vi "EnFlo_Error_Handler.vi"(3 "error in (no error)":errorcluster, 4 "Error Type":string, 5 "Dialog Box (T)":bool=TRUE) -> (0 "Continue":bool, 1 "SMS Message":string, 2 "Email Message":string)   [LabVIEW 2014]
uses:
  Controls/Post_Process.ctl
  <vilib>/Utility/error.llb/DialogType.ctl
  Globals/Meas_global.vi
  Globals/Trav_pos_global.vi
  Globals/Preference_global.vi
  Email_transfer_global.vi
  Globals/Dynamic_call_global.ph.vi
panel:
  out "error out":errorcluster
  in  "Case Constant\n(See Context Help)":bool
  out "Server copy Location":path
  out "Hours Running":dbl format="%.2f"
  out "Error Information":string
  out "Log Files":path[](array[path])
  out "Frequency":i32
  out "Error Analysis":string
  out "Error Types":string[](array[string])
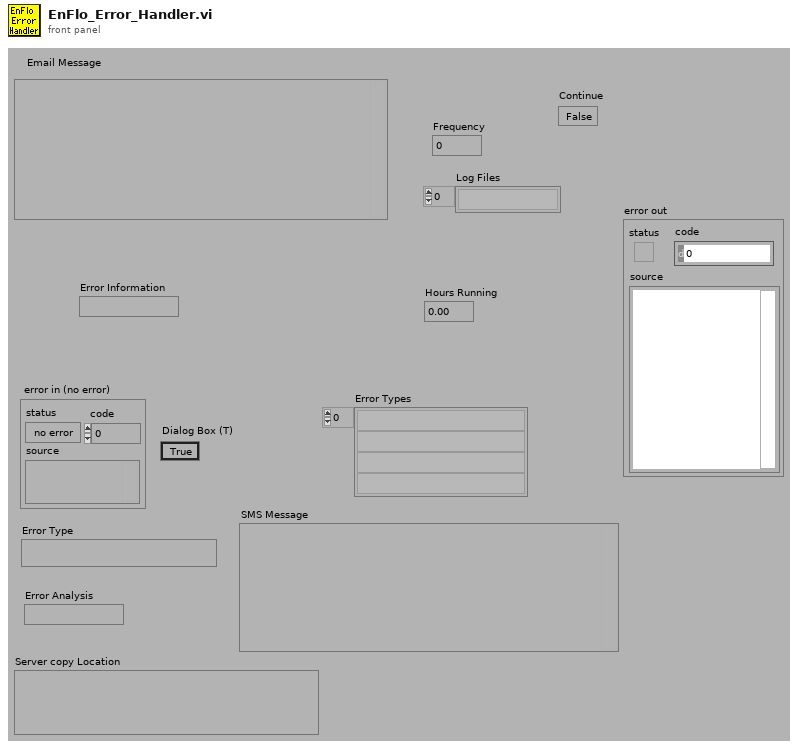
[diagram p1: front panel]
types:
  T1 = typedef "Post_Process.ctl" = enum16{"Take New Data", "Post Process Raw Data File"}
  T2 = cluster{"path":path, "data":string, "binary":bool, "MIME content-type \n(application/octet-stream)":string}[]
  T3 = typedef "DialogType.ctl" = u16
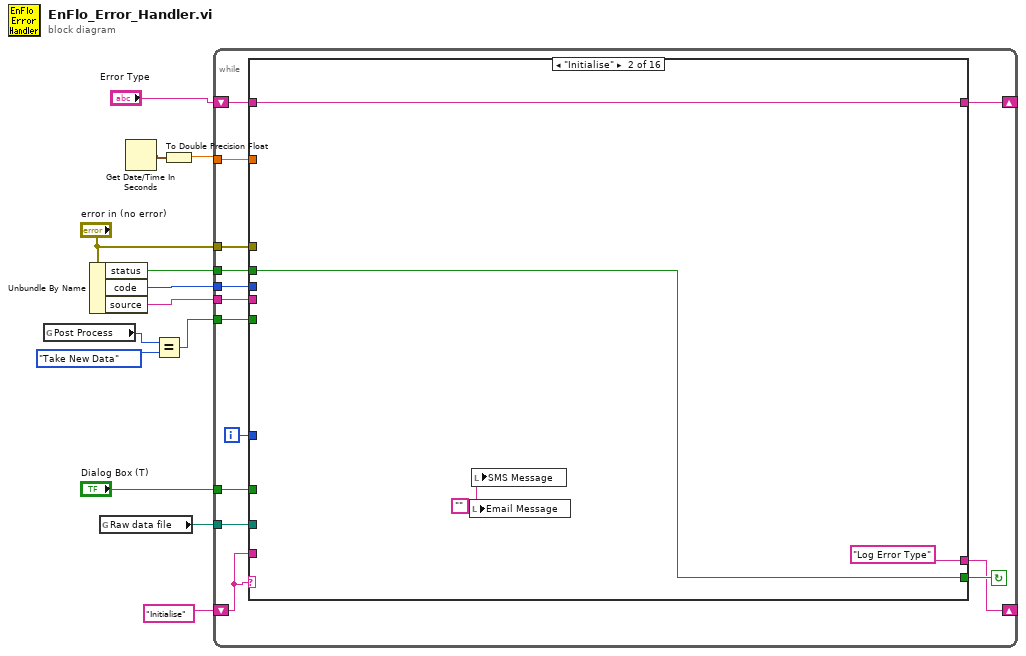
[diagram p0: block diagram]
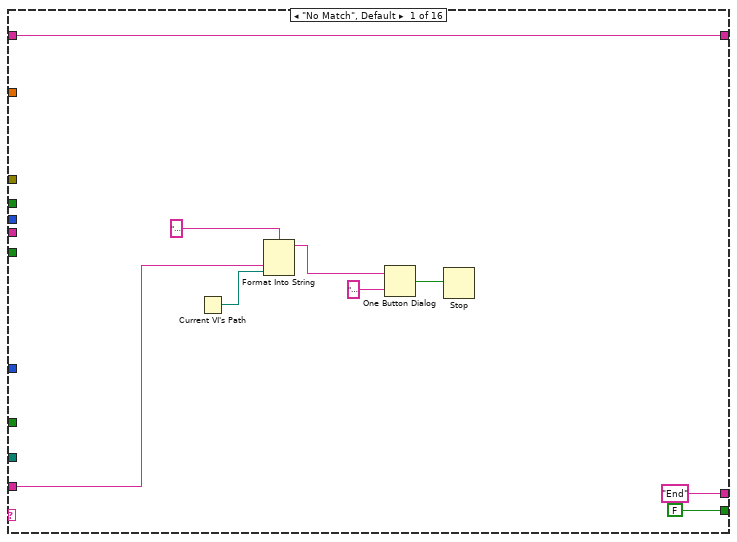
[diagram p2: hidden frame]
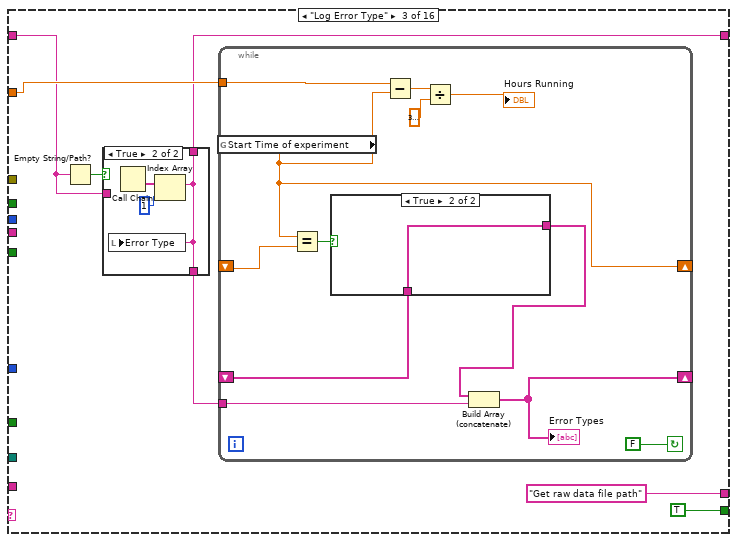
[diagram p3: hidden frame]
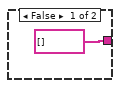
[diagram p4: hidden frame]
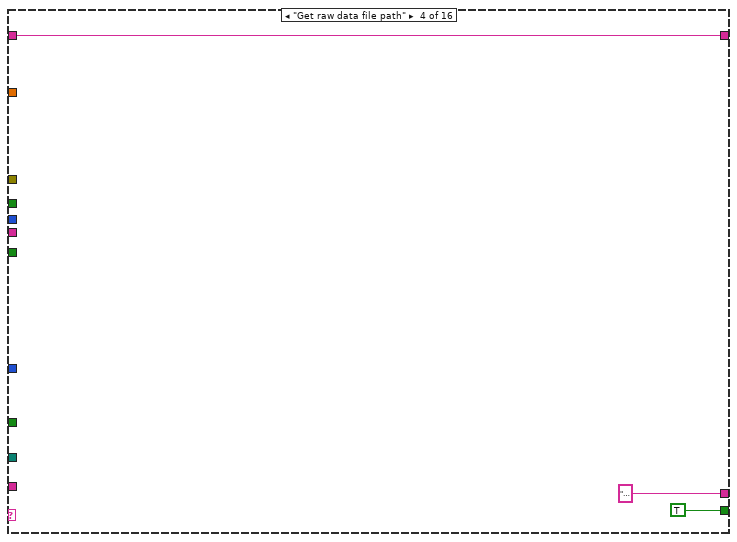
[diagram p6: hidden frame]
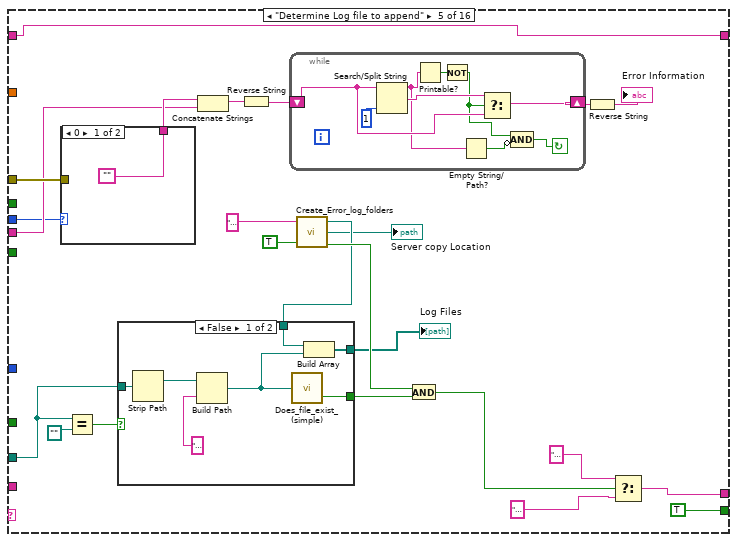
[diagram p7: hidden frame]
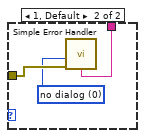
[diagram p8: hidden frame]
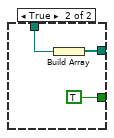
[diagram p9: hidden frame]
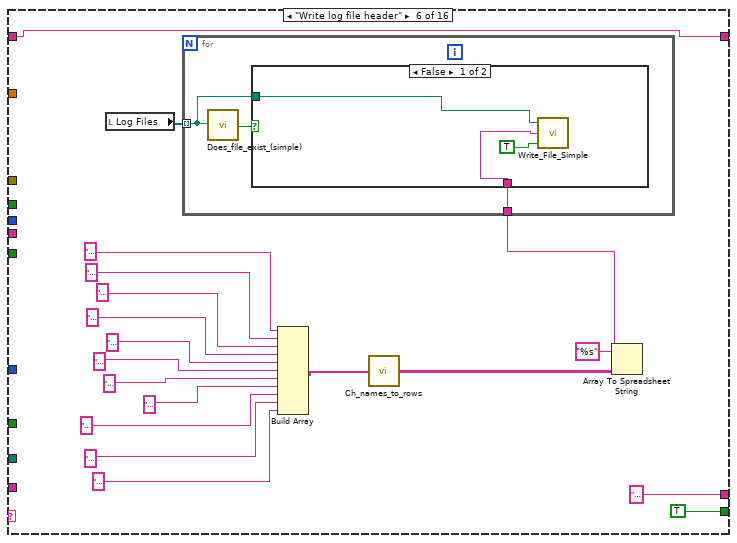
[diagram p10: hidden frame]
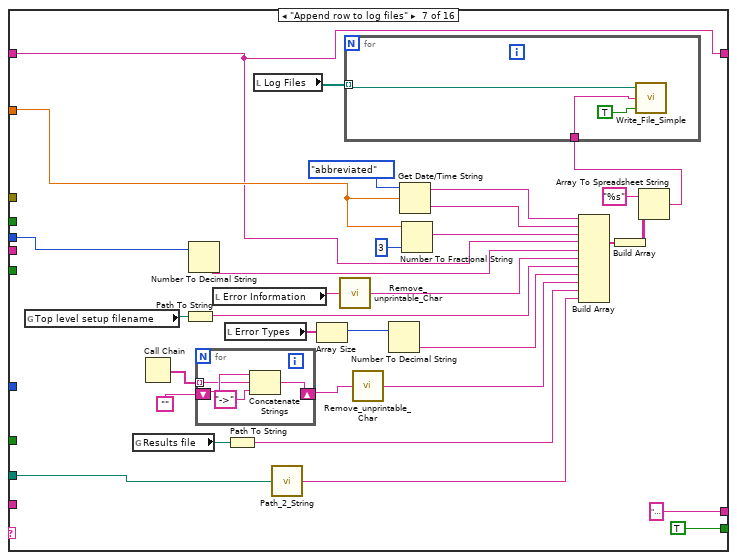
[diagram p12: hidden frame]
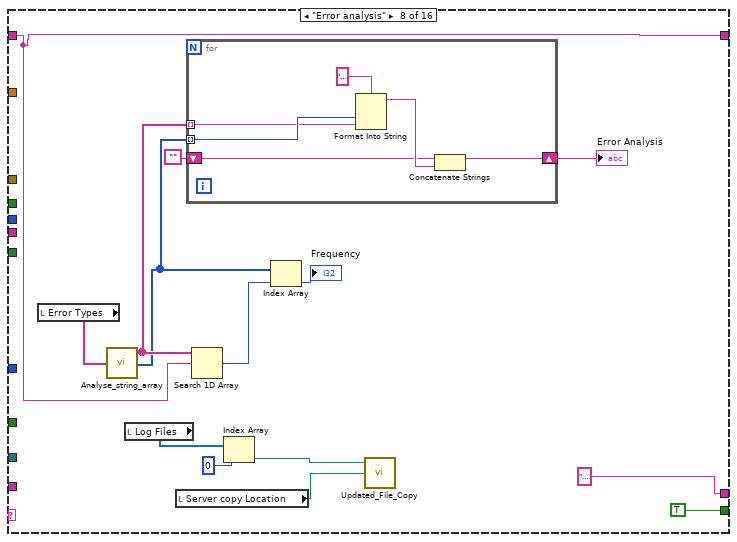
[diagram p13: hidden frame]
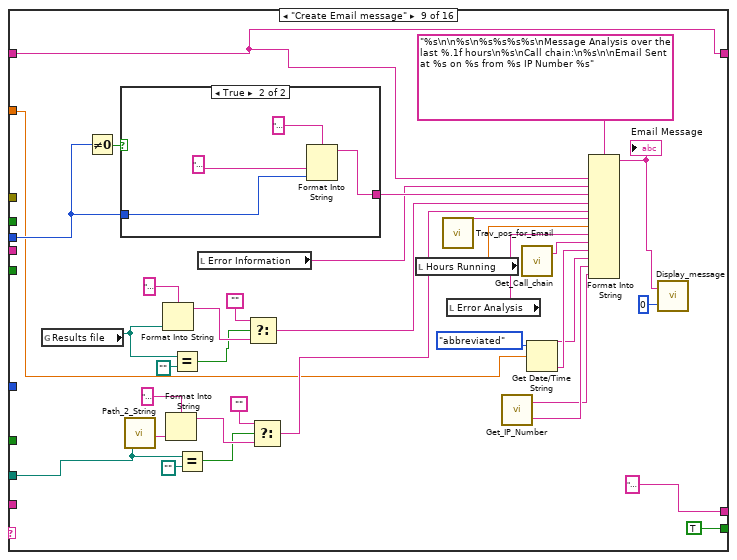
[diagram p14: hidden frame]
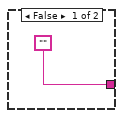
[diagram p15: hidden frame]
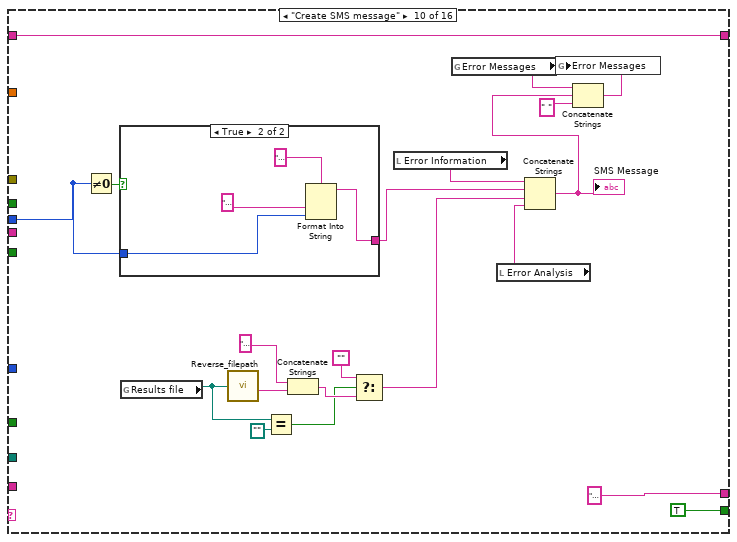
[diagram p16: hidden frame]
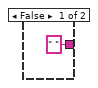
[diagram p17: hidden frame]
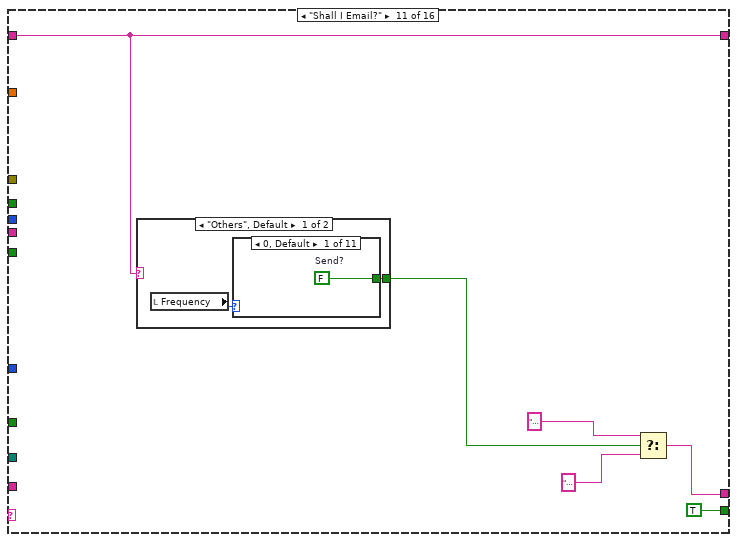
[diagram p18: hidden frame]
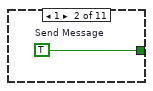
[diagram p19: hidden frame]
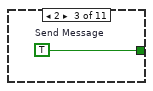
[diagram p20: hidden frame]
diagram:
  n1 = global read "Meas_global.vi" "Post Process"() -> (w6:T1)
  n2 = Unbundle By Name("error in (no error)") -> ("status"=w12:bool, "code"=w11:i32, "source"=w10:string)
  n3 = global read "Meas_global.vi" "Raw data file"() -> (w1:path)
  n4 = Get Date/Time In Seconds() -> (seconds since 1Jan1904=w9:timestamp)
  n5 = Equal?(x=w6, y=Post_Process."Take New Data" ("Post Process")) -> (x = y?=w4:bool)
  n6 = To Double Precision Float(number=w9) -> (double precision float=w13:dbl)
  n7 = while {
    tunnel: w10 -> [w21]
    tunnel: w11 -> [w23]
    tunnel: w12 -> [w24]
    tunnel: w13 -> [w25]
    shift-left: "Initialise" -> [w20]
    shift-right: [w26] -> _
    shift-right: [w18] -> _
    shift-left: "Error Type" -> [w19]
    tunnel: w4 -> [w17]
    tunnel: "Dialog Box (T)" -> [w16]
    tunnel: "error in (no error)" -> [w15]
    tunnel: w1 -> [w14]
    i -> [w22]
    stop <- w27 continue-if-true
    n8 = case shown="\"Initialise\"" w20 {
      tunnel: [FALSE ("Abort") w40 TRUE ("status") TRUE ("status") TRUE ("status") TRUE TRUE TRUE ("status") TRUE ("Abort") TRUE ("status") TRUE ("Abort") TRUE ("Abort") TRUE ("Abort") w335 w346 FALSE ("Abort")] -> w27
      tunnel: ["End" ("f") "Log Error Type" "Get raw data file path" ("f") "Determine Log file to append" ("f") w90 "Append row to log files" ("f") "Error analysis" ("f") "Create Email message" ("f") "Create SMS message" "Shall I Email?" w267 "Clear Email attachments" "Is ADAM scan table running?" ("f") "Show timed error dialog" "Stop" "End"] -> w26
      tunnel: w25 -> [_ _ w44 _ _ _ w146 _ w210 _ _ _ _ _ _ _]
      tunnel: w24 -> [_ w40 _ _ _ _ _ _ _ _ _ _ _ _ _ _]
      tunnel: w23 -> [_ _ _ _ w70 _ w166 _ w232 w257 _ _ _ _ _ _]
      tunnel: w22 -> [_ _ _ _ _ _ _ _ _ _ _ _ _ _ _ _]
      tunnel: w21 -> [_ _ _ _ w72 _ _ _ _ _ _ _ _ _ _ _]
      tunnel: w20 -> [w31 _ _ _ _ _ _ _ _ _ _ _ _ _ _ _]
      tunnel: w19 -> [w28 w37 w42 w66 w77 w116 w143 w184 w204 w239 w269 w287 w333 w337 w344 w350]
      tunnel: [w28 w37 w41 w66 w77 w116 w143 w184 w204 w239 w269 w287 w333 w337 w344 w350] -> w18
      tunnel: w17 -> [_ _ _ _ _ _ _ _ _ _ _ w284 _ _ _ _]
      tunnel: w16 -> [_ _ _ _ _ _ _ _ _ _ _ _ _ w334 _ _]
      tunnel: w15 -> [_ _ _ _ w74 _ _ _ _ _ _ _ _ _ _ _]
      tunnel: w14 -> [_ _ _ _ w69 _ w141 _ w199 _ _ _ _ _ _ _]
      frame "No Match", Default {
        n9 = Current VI's Path() -> (path=w32:path)
        n10 = Format Into String(format string="The Case\"%s\" was not Matched\nin VI named\n'%s\"" ("Format String"), w31, w32) -> (resulting string=w35:string)  [unwired: 2 in, 1 out]
        n11 = One Button Dialog(message=w35, button name ("OK")="STOP") -> (true=w33:bool)
        n12 = Stop(stop? (T)=w33) -> ()
      }
      frame "Initialise" {
        w39 = ""
        n13 = local write "Email Message"(w39) -> ()
        n14 = local write "SMS Message"(w39) -> ()
      }
      frame "Log Error Type" {
        n15 = Empty String/Path?(string/path=w42) -> (empty?=w46:bool)
        n16 = case shown="True" w46 {
          tunnel: [w62 w63] -> w45
          tunnel: w42 -> [w62 _]
          tunnel: [w62 w63] -> w41
          frame False {
          }
          frame True {
            n17 = Call Chain() -> (call chain=w65:string[])
            n18 = Index Array(array=w65, index=1 ("Index")) -> (element=w63:string)
            n19 = local write "Error Type"(w63) -> ()
          }
        }
        n20 = while {
          tunnel: w44 -> [w50]
          shift-left: _ -> [w57]
          shift-right: [w56] -> _
          shift-left: _ -> [w55]
          shift-right: [w53] -> _
          tunnel: w45 -> [w58]
          stop <- FALSE continue-if-true
          n21 = global read "Meas_global.vi" "Start Time of experiment"() -> (w53:dbl)
          n22 = Equal?(x=w53, y=w55) -> (x = y?=w54:bool)
          n23 = case shown="True" w54 {
            tunnel: [string[] [] w61] -> w59
            tunnel: w57 -> [_ w61]
            frame False {
            }
            frame True {
            }
          }
          n24 = Subtract(x=w50, y=w53) -> (x-y=w52:dbl)
          n25 = Divide(x=w52, y=3600.0) -> (x/y=→"Hours Running":dbl)
          n26 = Build Array (concatenate)(w59, w58) -> (w56:string[])
          "Error Types" <- w56
        }
      }
      frame "Get raw data file path" {
      }
      frame "Determine Log file to append" {
        n27 = case shown="0" w70 {
          tunnel: w74 -> [_ w96]
          tunnel: ["" w94] -> w73
          frame 0 {
          }
          frame 1, Default {
            w95 = T3 0 items=["no dialog", "OK message", "continue or stop message", "OK message + warnings", "continue/stop + warnings"] ("type of dialog (OK msg:1)")
            n28 = call <vilib>:"Simple Error Handler.vi"("type of dialog (OK msg:1)"=w95, "error in (no error)"=w96) -> ("message"=w94:string)  [unwired: 7 out]
          }
        }
        n29 = Equal?(x=w69, y=path "") -> (x = y?=w88:bool)
        n30 = Concatenate Strings(w73, w72) -> (w71:string)
        n31 = Reverse String(1:w71) -> (0:w82:string)
        n32 = while {
          shift-left: w82 -> [w103]
          shift-right: [w102] -> w81
          stop <- w97 continue-if-true
          n33 = Search/Split String(string=w103, offset (0)=1 ("length")) -> (substring before match=w100:string, match + rest of string=w104:string)  [unwired: 2 out]
          n34 = Printable?(1:w100) -> (0:w101:bool)
          n35 = Not(x=w101) -> (.not. x?=w99:bool)
          n36 = Empty String/Path?(string/path=w100) -> (empty?=w98:bool)
          n37 = Select(t=w104, s=w99, f=w103) -> (s? t:f=w102:string)
          n38 = Compound Arithmetic op=AND(w99, invert w98) -> (w97:bool)
        }
        n39 = call "Create_Error_log_folders.vi"("Per Day Log File?"=TRUE, "Log Filename"="Messages" ("Input Element")) -> ("exists?"=w86:bool, "Server copy Location"=→"Server copy Location":path, "Local Log File"=w84:path)  [unwired: 1 in]
        n40 = case shown="False" w88 {
          tunnel: w69 -> [w112 _]
          tunnel: [w109 TRUE ("exists?")] -> w87
          tunnel: w84 -> [w108 w114]
          tunnel: [w106 w113] -> w83
          frame False {
            n41 = Strip Path(path=w112) -> (stripped path=w111:path)  [unwired: 1 out]
            n42 = Build Path(base path=w111, name or relative path="Message_Log_File.xls") -> (appended path=w107:path)
            n43 = call "Does_file_exist_(simple).vi"("Pathname"=w107) -> ("exists?"=w109:bool)
            n44 = Build Array(w108, w107) -> (w106:path[])
          }
          frame True {
            n45 = Build Array(w114) -> (w113:path[])
          }
        }
        "Log Files" <- w83
        n46 = And(x=w86, y=w87) -> (x .and. y?=w85:bool)
        n47 = Reverse String(1:w81) -> (0:→"Error Information":string)
        n48 = Select(t="Append row to log files", s=w85, f="Write log file header") -> (s? t:f=w90:string)
      }
      frame "Write log file header" {
        n49 = local read "Log Files"() -> (w120:path[])
        n50 = Build Array("Date::", "Time::", "Seconds:Since:1st Jan 1904", "Error:Type:", "Labview:Error:Code", "Error:Description:", "Multi Run:Setup:Name", "Error Number:Since Start of:Multi Run Prog", "VI:Call:Chain", "Results:File:Path", "Raw Data:File:Path") -> (w119:string[])
        n51 = call "Ch_names_to_rows.vi"("Channel Names"=w119) -> ("3 Row names"=w118:string[][])
        n52 = Array To Spreadsheet String(array=w118, 3:"%s" ("format string")) -> (spreadsheet string=w124:string)  [unwired: 1 out]
        n53 = for {
          tunnel: w124 -> [w137]
          tunnel: w120 -> [w135] mode=indexing
          n54 = call "Does_file_exist_(simple).vi"("Pathname"=w135) -> ("exists?"=w136:bool)
          n55 = case shown="False" w136 {
            tunnel: w137 -> [w139 _]
            tunnel: w135 -> [w138 _]
            frame False {
              n56 = call "Write_File_Simple.vi"("append to file? (new file:F)"=TRUE, "character string"=w139, "file path"=w138) -> ()  [unwired: 2 out]
            }
            frame True {
            }
          }
        }
      }
      frame "Append row to log files" {
        n57 = global read "Trav_pos_global.vi" "Top level setup filename"() -> (w168:path)
        n58 = global read "Meas_global.vi" "Results file"() -> (w151:path)
        n59 = Call Chain() -> (call chain=w156:string[])
        n60 = Path To String(path=w168) -> (string=w163:string)
        n61 = Number To Decimal String(number=w166) -> (decimal integer string=w165:string)  [unwired: 1 out]
        n62 = for {
          shift-right: [w175] -> w155
          shift-left: "" -> [w178]
          tunnel: w156 -> [w177] mode=indexing
          n63 = Concatenate Strings(w178, w177, "->" ("Substring")) -> (w175:string)
        }
        n64 = local read "Error Information"() -> (w148:string)
        n65 = local read "Error Types"() -> (w161:string[])
        n66 = Path To String(path=w151) -> (string=w150:string)
        n67 = local read "Log Files"() -> (w149:path[])
        n68 = call "Path_2_String.vi"("Real Path"=w141) -> ("Path String"=w142:string)
        n69 = Array Size(array=w161) -> (size(s)=w167:i32)
        n70 = call "Remove_unprintable_Char.vi"("Input String"=w148) -> ("Output String"=w164:string)
        n71 = call "Remove_unprintable_Char.vi"("Input String"=w155) -> ("Output String"=w157:string)
        n72 = Number To Decimal String(number=w167) -> (decimal integer string=w162:string)  [unwired: 1 out]
        n73 = Get Date/Time String(date format (0)=enum16{"short", "long", "abbreviated"}."abbreviated", seconds (now)=w146) -> (date string=w170:string, time string=w169:string)  [unwired: 1 out]
        n74 = Number To Fractional String(number=w146, precision (6)=i16 3) -> (F-format string=w145:string)  [unwired: 2 out]
        n75 = Build Array(w170, w169, w145, w143, w165, w164, w163, w162, w157, w150, w142) -> (w152:string[])
        n76 = Build Array(w152) -> (w160:string[][])
        n77 = Array To Spreadsheet String(array=w160, 3:"%s" ("format string")) -> (spreadsheet string=w158:string)  [unwired: 1 out]
        n78 = for {
          tunnel: w158 -> [w173]
          tunnel: w149 -> [w172] mode=indexing
          n79 = call "Write_File_Simple.vi"("append to file? (new file:F)"=TRUE, "character string"=w173, "file path"=w172) -> ()  [unwired: 2 out]
        }
      }
      frame "Error analysis" {
        n80 = local read "Error Types"() -> (w187:string[])
        n81 = call "Analyse_string_array.vi"("String array"=w187) -> ("Unique strings"=w191:string[], "Frequency"=w190:i32[])  [unwired: 1 out]
        n82 = local read "Log Files"() -> (w182:path[])
        n83 = local read "Server copy Location"() -> (w179:path)
        n84 = for {
          tunnel: w191 -> [w196] mode=indexing
          tunnel: w190 -> [w197] mode=indexing
          shift-right: [w193] -> w188
          shift-left: "" -> [w194]
          n85 = Format Into String(format string="%d %s\n" ("Format String"), w197, w196) -> (resulting string=w195:string)  [unwired: 2 in, 1 out]
          n86 = Concatenate Strings(w194, w195) -> (w193:string)
        }
        "Error Analysis" <- w188
        n87 = Search 1D Array(1D array=w191, element=w184) -> (index of element=w192:i32)  [unwired: 1 out]
        n88 = Index Array(array=w182, index=0) -> (element=w180:path)
        n89 = Index Array(array=w190, index=w192) -> (element=→"Frequency":i32)
        n90 = call "Updated_File_Copy.vi"("Target Path"=w179, "Source Path"=w180) -> ()  [unwired: 2 out]
      }
      frame "Create Email message" {
        n91 = global read "Meas_global.vi" "Results file"() -> (w217:path)
        n92 = Not Equal To 0?(x=w232) -> (x != 0?=w233:bool)
        n93 = case shown="True" w233 {
          tunnel: w232 -> [_ w237]
          tunnel: ["" w235] -> w231
          frame False {
          }
          frame True {
            n94 = Format Into String(format string="%s %d\n" ("Format String"), "Having the error code ", w237) -> (resulting string=w235:string)  [unwired: 2 in, 1 out]
          }
        }
        n95 = call "Path_2_String.vi"("Real Path"=w199) -> ("Path String"=w202:string)
        n96 = Format Into String(format string="\\nResults File:\\n%s\\n" ("Format String"), w217) -> (resulting string=w223:string)  [unwired: 2 in, 1 out]
        n97 = Format Into String(format string="\\nRaw Data File:\\n%s\\n" ("Format String"), w202) -> (resulting string=w221:string)  [unwired: 2 in, 1 out]
        n98 = Equal?(x=w217, y=path "") -> (x = y?=w216:bool)
        n99 = Equal?(x=w199, y=path "") -> (x = y?=w218:bool)
        n100 = local read "Error Information"() -> (w215:string)
        n101 = Select(t="", s=w216, f=w223) -> (s? t:f=w226:string)
        n102 = Select(t="", s=w218, f=w221) -> (s? t:f=w225:string)
        n103 = local read "Hours Running"() -> (w213:dbl)
        n104 = call "Trav_pos_for_Email.vi"() -> ("String"=w214:string)
        n105 = local read "Error Analysis"() -> (w212:string)
        n106 = call "Get_IP_Number.vi"() -> ("Computer Name"=w201:string, "IP Number"=w200:string)
        n107 = call "Get_Call_chain.vi"() -> ("Output String"=w211:string)  [unwired: 1 in, 1 out]
        n108 = Get Date/Time String(date format (0)=enum16{"short", "long", "abbreviated"}."abbreviated", seconds (now)=w210) -> (date string=w206:string, time string=w208:string)  [unwired: 1 out]
        n109 = Format Into String(format string="%s\n\n%s\n%s%s%s%s\nMessage Analysis over the last %.1f hours\n%s\nCall chain:\n%s\n\nEmail Sent at %s on %s from %s IP Number %s" ("Format String"), w204, w215, w231, w226, w225, w214, w213, w212, w211, w208, w206, w201, w200) -> (resulting string=w207:string)  [unwired: 2 in, 1 out]
        "Email Message" <- w207
        n110 = call "Display_message.vi"("Time to display message"=u32 0, "Message"=w207) -> ()  [unwired: 2 out]
      }
      frame "Create SMS message" {
        n111 = Not Equal To 0?(x=w257) -> (x != 0?=w258:bool)
        n112 = case shown="True" w258 {
          tunnel: w257 -> [_ w262]
          tunnel: [" " w260] -> w256
          frame False {
          }
          frame True {
            n113 = Format Into String(format string="%s %d, " ("Format String"), " err code ", w262) -> (resulting string=w260:string)  [unwired: 2 in, 1 out]
          }
        }
        n114 = global read "Meas_global.vi" "Results file"() -> (w243:path)
        n115 = call "Reverse_filepath.vi"("Filename"=w243) -> ("Reversed Filepath"=w250:string)
        n116 = Equal?(x=w243, y=path "") -> (x = y?=w242:bool)
        n117 = Concatenate Strings("File: ", w250) -> (w248:string)
        n118 = Select(t="", s=w242, f=w248) -> (s? t:f=w246:string)
        n119 = local read "Error Information"() -> (w241:string)
        n120 = global read "Meas_global.vi" "Error Messages"() -> (w253:string)
        n121 = local read "Error Analysis"() -> (w245:string)
        n122 = Concatenate Strings(w241, w256, w246, w245) -> (w251:string)
        "SMS Message" <- w251
        n123 = Concatenate Strings(w253, w251, " ") -> (w252:string)
        n124 = global write "Meas_global.vi" "Error Messages"(w252) -> ()
      }
      frame "Shall I Email?" {
        n125 = case shown="\"Others\", Default" w269 {
          tunnel: [w270 TRUE ("Send Message")] -> w268
          frame "Others", Default {
            n126 = local read "Frequency"() -> (w271:i32)
            n127 = case shown="0, Default" w271 {
              tunnel: [w272 w273 w274 w275 TRUE TRUE TRUE TRUE TRUE TRUE w282] -> w270
              frame 0, Default {
                w272 = FALSE  # Send?
              }
              frame 1 {
                w273 = TRUE  # Send Message
              }
              frame 2 {
                w274 = TRUE  # Send Message
              }
              frame 5 {
                w275 = TRUE  # Send Message
              }
              frame 10 {
              }
              frame 20 {
              }
              frame 50 {
              }
              frame 100 {
              }
              frame 200 {
              }
              frame 500 {
              }
              frame 1000 {
                w282 = TRUE  # Send Message
              }
            }
          }
          frame "Message" {
          }
        }
        n128 = Select(t="Send Emails etc", s=w268, f="Clear Email attachments") -> (s? t:f=w267:string)
      }
      frame "Send Emails etc" {
        n129 = global read "Preference_global.vi" "LabVIEW Administrators"() -> (w285:string[])
        n130 = case shown="True" w284 {
          tunnel: w287 -> [_ w290]
          tunnel: w285 -> [_ w289]
          frame False {
          }
          frame True {
            n131 = stacked-sequence {
              tunnel: w290 -> [_ w295 _ _ w317]
              tunnel: w289 -> [w292 _ w309 _ _]
              frame #0 {
                n132 = global read "Meas_global.vi" "People to Email"() -> (w291:string[])
                n133 = global read "Email_transfer_global.vi" "recipients"() -> (w293:string[])
                n134 = Build Array (concatenate)(w293, w292, w291) -> (w294:string[])
                n135 = global write "Email_transfer_global.vi" "recipients"(w294) -> ()
              }
              frame #1 {
                n136 = global write "Email_transfer_global.vi" "subject ([No Subject])"(w295) -> ()
              }
              frame #2 {
                n137 = local read "Email Message"() -> (w296:string)
                n138 = Concatenate Strings(w296, "\nThis email has been generated  automatically by LabVIEW. If you need help with understanding the email, or want to be removed from the mailing list please contact:\n") -> (w307:string)
                n139 = Concatenate Strings(" or ", "\r\n") -> (w303:string)
                n140 = for {
                  shift-right: [w311] -> w306
                  shift-left: w307 -> [w313]
                  tunnel: w309 -> [w312] mode=indexing
                  tunnel: w303 -> [w310]
                  n141 = Concatenate Strings(w313, w312, w310) -> (w311:string)
                }
                n142 = String Length(string=w303) -> (length=w301:i32)
                n143 = String Length(string=w306) -> (length=w302:i32)
                n144 = Subtract(x=w302, y=w301) -> (x-y=w300:i32)
                n145 = String Subset(string=w306, length (rest)=w300) -> (substring=w299:string)  [unwired: 1 out]
                n146 = Concatenate Strings(w299, "\r\n") -> (w297:string)
                n147 = global write "Email_transfer_global.vi" "message"(w297) -> ()
              }
              frame #3 {
                n148 = call "Launch_Async_Email.vi"() -> ("error out"=→"error out":errorcluster)  [unwired: 2 out]
              }
              frame #4 {
                n149 = local read "Frequency"() -> (w315:i32)
                n150 = case shown="\"No Match\", Default" w317 {
                  tunnel: [TRUE FALSE w325 FALSE] -> w319
                  tunnel: w315 -> [_ _ w327 _]
                  frame "No Match", Default {
                  }
                  frame "Pulse Width Error" {
                  }
                  frame "LDA Invalid Bursts" {
                    n151 = Greater?(x=w327, y=4) -> (0:w325:bool)
                  }
                  frame "Warning" {
                  }
                }
                n152 = global read "Meas_global.vi" "People to Email"() -> (w316:string[])
                n153 = local read "SMS Message"() -> (w318:string)
                n154 = case shown="True" w319 {
                  tunnel: w318 -> [_ w322]
                  tunnel: w316 -> [_ w321]
                  tunnel: w317 -> [_ w320]
                  frame False {
                  }
                  frame True {
                    n155 = call "SMS_to_mobile.vi"("SMS address"=w321, "Subject"=w320, "Message"=w322) -> ()  [unwired: 3 out]
                  }
                }
              }
            }
          }
        }
      }
      frame "Clear Email attachments" {
        n156 = global write "Email_transfer_global.vi" "attachments"(T2 [] ("attachments")) -> ()
        n157 = global write "Email_transfer_global.vi" "recipients"(string[] [] ("recipients")) -> ()
      }
      frame "Is ADAM scan table running?" {
        n158 = Open VI Reference(vi path="ADAM_scan_table.vi") -> (vi reference=w341:refnum<vi>, error out=w340:errorcluster)  [unwired: 1 in, 4 out]
        n159 = Unbundle By Name(w340) -> ("status"=w336:bool)
        n160 = case shown="False" w336 {
          tunnel: w340 -> [w343 _]
          tunnel: w341 -> [w342 _]
          frame False {
            n161 = Close Reference(reference=w342, error in (no error)=w343) -> ()  [unwired: 1 out]
          }
          frame True {
          }
        }
        n162 = Compound Arithmetic op=AND(w336, w334) -> (w335:bool)
      }
      frame "Show timed error dialog" {
        n163 = local read "Email Message"() -> (w348:string)
        n164 = call "Timed_Error_dialog.vi"("Message"=w348, "Seconds to wait"=60.0) -> ("Ignore"=→"Continue":bool, "Abort"=w346:bool)
      }
      frame "Stop" {
        n165 = stacked-sequence {
          seq-local: [_ w360 _ _ _] -> [_ _ w374 _ _]
          frame #0 {
            n166 = call "Program_Active_Aborting.vi"() -> ()  [unwired: 6 out]
          }
          frame #1 {
            n167 = Build Array("Edit_BSA_setup.vi", "Measurement_input_panel.vi", "Input_Value_Dialog.vi", "Input_String_Dialog.vi", "Calibration_user_input.vi", "Input_Traverse_position.vi", "User_Metadata.vi", "Preference_Panel.vi", "Traverse_Space.vi", "Enter_Temp_Press.vi", "EnFlo_Tunnel_Setup.vi", "Gas_Setup.vi", "Correlation_Display.vi", "Serial_Setup.vi", "Port_Names.vi", "Select_Strings.vi", "Edit_Template_File.vi", "Select_a_Channel.vi", "Output_file_Panel.vi", "Enter_LDA_Setup.vi") -> (w360:string[])
          }
          frame #2 {
            n168 = for {
              tunnel: w374 -> [w375] mode=indexing
              n169 = Open VI Reference(vi path=w375) -> (vi reference=w380:refnum<vi>, error out=w379:errorcluster)  [unwired: 1 in, 4 out]
              n170 = property class="VI"(reference=w380, error in=w379, "Front Panel Window:Open"=FALSE) -> (reference out=w378:refnum<vi>, error out=w377:errorcluster)
              n171 = Close Reference(reference=w378, error in (no error)=w377) -> ()  [unwired: 1 out]
            }
          }
          frame #3 {
            n172 = case shown="True" "Case Constant\n(See Context Help)" {
              frame False {
              }
              frame True {
                # "Cased out 4/7/07 because it hung code"
                n173 = global write "Dynamic_call_global.ph.vi" "EnFlo Hub running?"(FALSE ("EnFlo Hub running?")) -> ()
              }
            }
          }
          frame #4 {
            n174 = Stop(stop? (T)=TRUE) -> ()
          }
        }
      }
    }
  }
